vi "calc mods from center.vi"(8 "error in (no error)":errorcluster, 11 "pivot center":T1 {"Y" format="%.4g"; "X" format="%.4g"}) -> (0 "error out":errorcluster)   [LabVIEW 2023]
uses:
  ctrl defs/ctrl XY coord.ctl
  ctrl defs/ctrl swerve module.ctl
  Global odometry.vi
panel:
  out "PARKING angle (deg)":dbl
  out "output to swerve module data":T2[](array[typedef]) {"corner wt (lbm)" format="%#.3f"; "POS" format="%.3g"; "coord wrt geom CTR"."Y" format="%.4g"; "coord wrt geom CTR"."X" format="%.4g"; "from pivot to module"."theta park (deg)" format="%.4g"; "from pivot to module"."theta spin (deg)" format="%.4g"; "from pivot to module"."theta (deg)" format="%.4g"; "from pivot to module"."R" format="%.4g"; "ABS" format="%.3g"; "target" format="%.3g"; "V" format="%.3g"}
  out "gem ctr to module":cluster{"geomX":dbl, "geomY":dbl}[](array[cluster])
  out "pivot to module":T1[](array[typedef]) {"Y" format="%.4g"; "X" format="%.4g"}
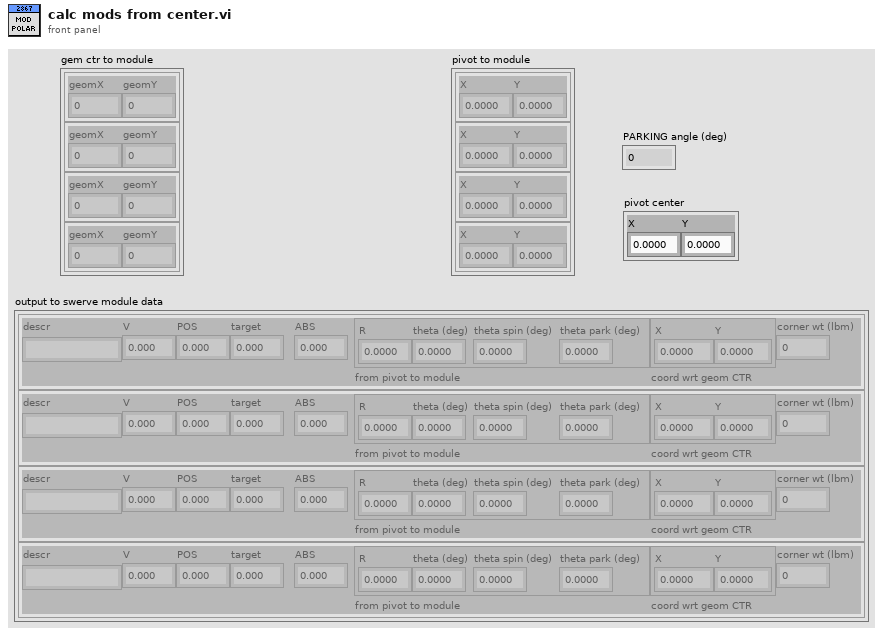
[diagram p1: front panel]
types:
  T1 = typedef "ctrl XY coord.ctl" = cluster{"X":dbl, "Y":dbl}
  T2 = typedef "ctrl swerve module.ctl" = cluster{"descr":string, "V":dbl, "POS":dbl, "target":dbl, "ABS":dbl, "from pivot to module":cluster{"R":dbl, "theta (deg)":dbl, "theta spin (deg)":dbl, "theta park (deg)":dbl}, "coord wrt geom CTR":cluster{"X":dbl, "Y":dbl}, "corner wt (lbm)":dbl}
  T3 = typedef "ctrl PARKING constants.ctl" = cluster{"angle (deg)":dbl, "%VBus":dbl}
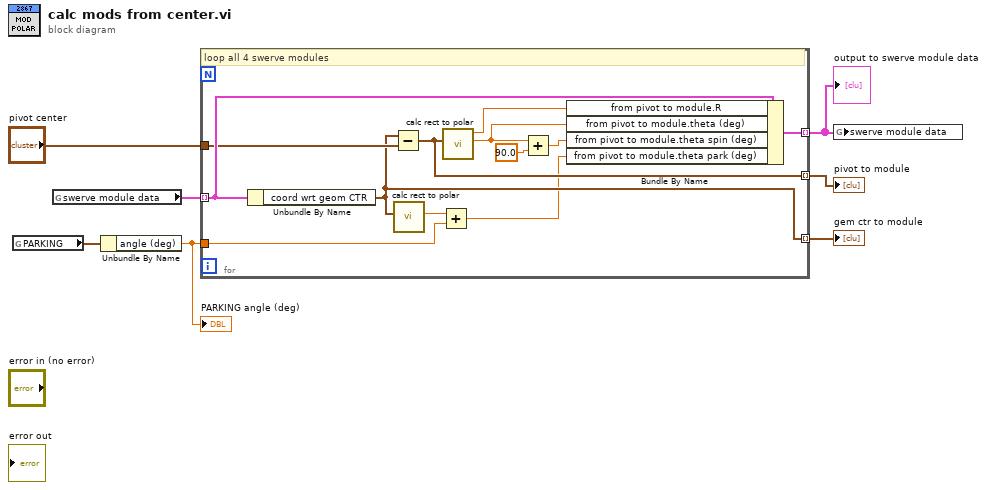
[diagram p0: block diagram]
diagram:
  n1 = global read "Global odometry.vi" "PARKING"() -> (w2:T3)
  n2 = global read "Global odometry.vi" "swerve module data"() -> (w7:T2[])
  n3 = Unbundle By Name(w2) -> ("angle (deg)"=w1:dbl)
  "PARKING angle (deg)" <- w1
  n4 = for {
    tunnel: w7 -> [w18] mode=indexing
    tunnel: [w19] -> w6 mode=indexing
    tunnel: "pivot center" -> [w15]
    tunnel: [w16] -> w5 mode=indexing
    tunnel: [w11] -> w4 mode=indexing
    tunnel: w1 -> [w8]
    # "loop all 4 swerve modules"
    n5 = Unbundle By Name(w18) -> ("coord wrt geom CTR"=w11:cluster{"X":dbl, "Y":dbl})
    n6 = Subtract(x=w11, y=w15) -> (x-y=w16:T1)
    n7 = call "calc rect to polar.vi"("XY"=w11) -> ("angle (deg)"=w10:dbl)  [unwired: 8 in, 2 out]
    n8 = Add(x=w10, y=w8) -> (x+y=w9:dbl)
    n9 = call "calc rect to polar.vi"("XY"=w16) -> ("angle (deg)"=w14:dbl, "Magnitude"=w17:dbl)  [unwired: 8 in, 1 out]
    n10 = Add(x=w14, y=90.0) -> (x+y=w13:dbl)
    n11 = Bundle By Name(cluster=w18, "from pivot to module.R"=w17, "from pivot to module.theta (deg)"=w14, "from pivot to module.theta spin (deg)"=w13, "from pivot to module.theta park (deg)"=w9) -> (w19:T2)
  }
  "pivot to module" <- w5
  "gem ctr to module" <- w4
  "output to swerve module data" <- w6
  n12 = global write "Global odometry.vi" "swerve module data"(w6) -> ()
